vi "Get Class Name.vi"(3 "lvclass":refnum<class>) -> (4 "Full Name":string, 5 "Child Name":string)   [LabVIEW 2016]
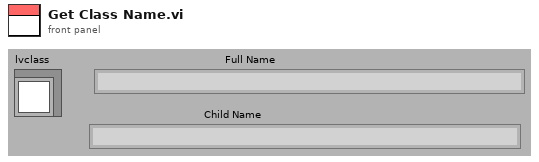
[diagram p1: front panel]
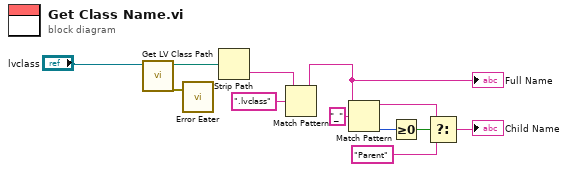
[diagram p0: block diagram]
diagram:
  n1 = call <vilib>:"Get LV Class Path.vi"("object"="lvclass") -> ("error out"=w3:errorcluster, "class path"=w2:path)  [unwired: 9 in]
  n2 = call "Error Eater.vi"("error in (no error)"=w3) -> ()  [unwired: 2 in]
  n3 = Strip Path(path=w2) -> (name=w1:string)  [unwired: 1 out]
  n4 = Match Pattern(string=w1, regular expression=".lvclass") -> (before substring=w5:string)  [unwired: 1 in, 3 out]
  "Full Name" <- w5
  n5 = Match Pattern(string=w5, regular expression="_") -> (before substring=w11:string, offset past match=w9:i32)  [unwired: 1 in, 2 out]
  n6 = Greater Or Equal To 0?(x=w9) -> (x >= 0?=w8:bool)
  n7 = Select(t=w11, s=w8, f="Parent") -> (s? t:f=→"Child Name":string)
